vi "ThermalMap.vi"() -> ()   [LabVIEW 2017]
uses:
  <vilib>/Utility/file.llb/Write Delimited Spreadsheet (I64).vi
panel:
  in  "Tab Control":enum32{"File", "Page 2"}(tab)
  in  "base path":path=path "E:/Materials Testing"
  in  "Filename":string="Run 0_image"
  out "file path":path=path "M:/Oceanoptics/TDMS test/Spectrometer.csv"
  out "output cluster":cluster{"Image Pixels (U8)":u8[][]}
  in  "Stop":bool
  out "Image Out":T1(plugin-control)
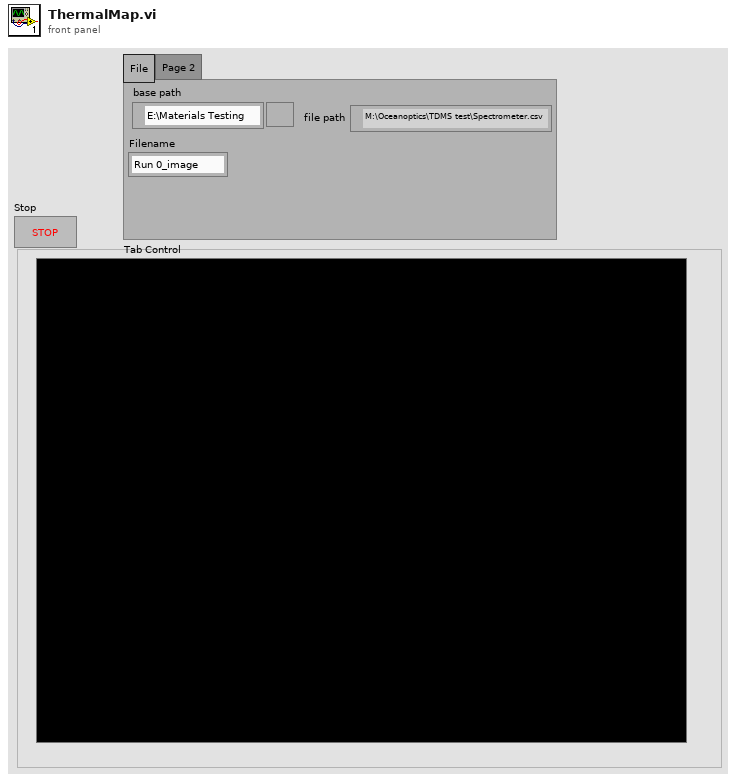
[diagram p1: front panel]
types:
  T1 = typedef "IMAQ Image.ctl" = refnum<image>
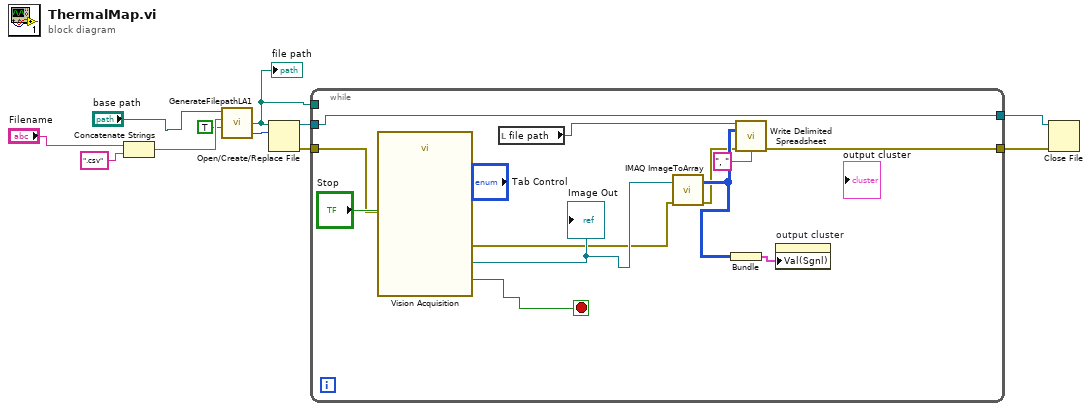
[diagram p0: block diagram]
diagram:
  n1 = Concatenate Strings("Filename", ".csv") -> (w7:string)
  n2 = call "GenerateFilepathLA1.vi"("Auto Date folder"=TRUE, "Filename"=w7, "base path"="base path") -> ("Numeric"=w9:i32, "file path"=w6:path)  [unwired: 1 in, 1 out]
  "file path" <- w6
  n3 = Open/Create/Replace File(file path (use dialog)=w6, operation (0:open)=w9) -> (refnum out=w5:refnum<file>, error out=w3:errorcluster)  [unwired: 4 in, 1 out]
  n4 = while {
    tunnel: w6 -> [_]
    tunnel: w5 -> [w16]
    tunnel: [w16] -> w4
    tunnel: w3 -> [w15]
    tunnel: [w12] -> w2
    stop <- w23 stop-if-true
    n5 = call "Vision Acquisition"("Stop (F)"="Stop", "error in"=w15) -> ("Image Out"=w21:T1, "Stopped"=w23:bool, "error out"=w14:errorcluster)  [unwired: 23 in]
    "Image Out" <- w21
    n6 = local read "file path"() -> (w18:path)
    n7 = call "IMAQ ImageToArray"("error in (no error)"=w14, "Image"=w21) -> ("error out"=w13:errorcluster, "Image Pixels (U8)"=w19:u8[][])  [unwired: 2 in, 3 out]
    n8 = Bundle("Image Pixels (U8)"=w19) -> (w20:cluster{"Image Pixels (U8)":u8[][]})  [unwired: 1 in]
    n9 = call-poly <vilib>:"Write Delimited Spreadsheet.vi"("file path (dialog if empty)"=w18, "2D data"=w19, "error in (no error)"=w13, "delimiter (\\t)"=", " ("delimiter (\\t)")) -> ("error out"=w12:errorcluster)  [unwired: 10 in, 1 out]
    n10 = property on="output cluster" class="Clust (strict)"("Val(Sgnl)"=w20) -> ()  [unwired: 2 in, 2 out]
  }
  n11 = Close File(refnum=w4, error in=w2) -> ()  [unwired: 2 out]
